vi "Split text segments from line.vi"(2 "Input line string":string) -> (16 "Text segments":string[](array[string]))   [LabVIEW 2020]
doc: "This VI returns single lines from input string. If number of lines (Array size) is known, algorithm is faster, otherwise Array size = 0 should be used. Sub-VI for VST?.vi and Define macro contents (with or without) delay.vi."
uses:
  <vilib>/regexp/Match Regular Expression.xnode
panel:
  # "Split line with tabs into text segments."
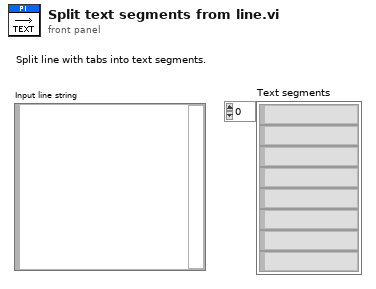
[diagram p1: front panel]
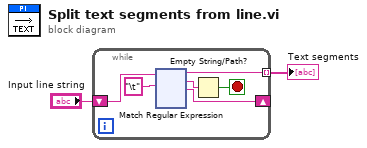
[diagram p0: block diagram]
diagram:
  n1 = while {
    shift-right: [w8] -> _
    shift-left: "Input line string" -> [w4]
    tunnel: [w7] -> w1 mode=indexing
    stop <- w5 stop-if-true
    n2 = xnode "Match Regular Expression"("input string"=w4, "regular expression"="\t") -> ("before match"=w7:string, "whole match"=w6:string, "after match"=w8:string)  [unwired: 4 in, 2 out]
    n3 = Empty String/Path?(string/path=w6) -> (empty?=w5:bool)
  }
  "Text segments" <- w1
